vi "crc16-ccitt.vi"(5 "Message":string, 11 "error in (no error)":errorcluster) -> (6 "CRC":i32 format="%x", 15 "error out":errorcluster)   [LabVIEW 2016]
doc: "This VI computes the CRC16 CCITT of any message. This implementation was derived from the C code provided by http://www.joegeluso.com/software/articles/ccitt.htm"
panel:
  out "Message  2":string
  # "POLY 1021"
  # "Initial Value = FFFF"
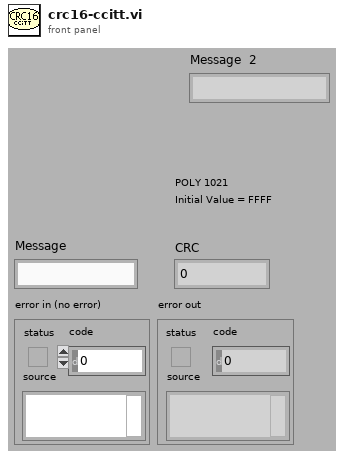
[diagram p1: front panel]
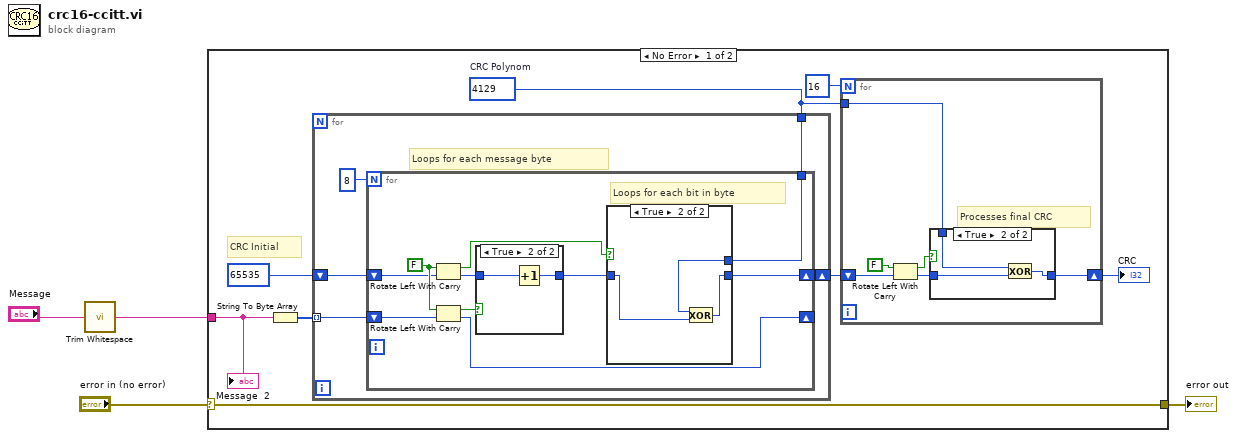
[diagram p0: block diagram]
diagram:
  n1 = call <vilib>:"Trim Whitespace.vi"("string"="Message") -> ("trimmed string"=w1:string)  [unwired: 1 in]
  n2 = case shown="No Error" "error in (no error)" {
    selector: "error in (no error)" -> [w7 w45]
    tunnel: [w7 w45] -> w3
    tunnel: w1 -> [w5 _]
    frame No Error {
      w6 = u16 4129  # CRC Polynom
      # "CRC Initial"
      n3 = String To Byte Array(string=w5) -> (unsigned byte array=w8:u8[])
      n4 = for {
        tunnel: w8 -> [w26] mode=indexing
        shift-right: [w24] -> w10
        shift-left: u16 65535 -> [w25]
        tunnel: w6 -> [w23]
        # "Loops for each message byte"
        n5 = for {
          N: 8 -> [_]
          shift-right: [w32] -> _
          shift-left: w26 -> [w31]
          shift-right: [w29] -> w24
          shift-left: w25 -> [w30]
          tunnel: w23 -> [w28]
          w33 = FALSE ("carry")
          # "Loops for each bit in byte"
          n6 = Rotate Left With Carry(2:w30, 3:w33) -> (0:w36:u16, 1:w37:bool)
          n7 = Rotate Left With Carry(2:w31, 3:w33) -> (0:w32:u8, 1:w34:bool)
          n8 = case shown="True" w34 {
            tunnel: [w38 w39] -> w35
            tunnel: w36 -> [w38 w40]
            frame False {
            }
            frame True {
              n9 = Increment(x=w40) -> (x+1=w39:u16)
            }
          }
          n10 = case shown="True" w37 {
            tunnel: w35 -> [w41 w44]
            tunnel: [w41 w43] -> w29
            tunnel: w28 -> [_ w42]
            frame False {
            }
            frame True {
              n11 = Exclusive Or(1:w44, 2:w42) -> (0:w43:u16)
            }
          }
        }
      }
      n12 = for {
        N: 16 -> [_]
        shift-right: [w16] -> w9
        shift-left: w10 -> [w15]
        tunnel: w6 -> [w13]
        # "Processes final CRC"
        n13 = Rotate Left With Carry(2:w15, 3:FALSE ("carry")) -> (0:w14:u16, 1:w18:bool)
        n14 = case shown="True" w18 {
          tunnel: w14 -> [w19 w21]
          tunnel: [w19 w22] -> w16
          tunnel: w13 -> [_ w20]
          frame False {
          }
          frame True {
            n15 = Exclusive Or(1:w21, 2:w20) -> (0:w22:u16)
          }
        }
      }
      "CRC" <- w9
      "Message  2" <- w5
    }
    frame Error {
    }
  }
  "error out" <- w3
